vi "CODMn停止命令 (子VI).vi"   [LabVIEW 2016, in "斯坦道CODMn.lvlib"]
uses:
  <vilib>/Plasmionique/MB Master/MB_Master_Serial/MB_Master_Serial.lvclass
  F:/Program Files/National Instruments/LabVIEW 2016/vi.lib/Plasmionique/MB Master/MB_Master/MB_Master.lvclass
  <vilib>/Plasmionique/MB Master/MB Master.lvlib
types:
  T1 = cluster{"baud rate (bps)":u32, "stop bits":u16, "parity":u16, "flow control":u16, "timeout":u32, "retries":i32}
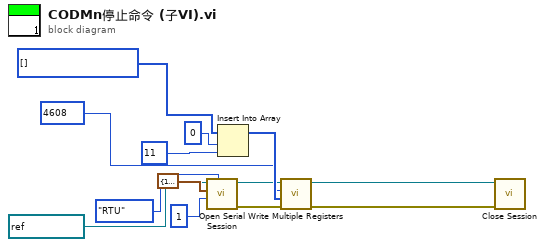
[diagram p0: block diagram]
diagram:
  n1 = call <vilib>:"Open Serial Session.vi"("Mode (RTU)"=enum16{"RTU", "ASCII"}."RTU", "Slave ID"=u8 1, "Serial Config"=T1 {"baud rate (bps)"=115200, "stop bits"=10, "parity"=0, "flow control"=0, "timeout"=1000, "retries"=1}, "VISA Resource"=refnum<visa-resource-name> "COM4") -> ("Error out"=w13:errorcluster, "MB_Serial session"=w3:refnum<class "MB_Master_Serial.lvclass">)  [unwired: 6 in]
  n2 = Insert Into Array(array=u16[] [] ("values"), index=0 ("索引"), new element=u16 11 ("address")) -> (w12:u16[])
  n3 = call <vilib>:"Write Multiple Registers.vi"("error in (no error)"=w13, "values"=w12, "starting address"=u16 4608 ("address"), "MB session in"=w3) -> ("error out"=w1:errorcluster, "MB session out"=w2:refnum<class "MB_Master_Serial.lvclass">)  [unwired: 6 in]
  n4 = call-dynamic "Close Session.vi"("error in (no error)"=w1, "MB_Serial session"=w2) -> ()  [unwired: 9 in, 1 out]
